vi "Set Aircraft GPS.vi"(7 "Aircraft ID":u8, 8 "Error In":errorcluster, 11 "Aircraft Att Data IN":T1) -> (0 "Error Out":errorcluster, 3 "Aircraft Att Data Out":T1)   [LabVIEW 2014]
uses:
  Controls/Aircraft GPS Data.ctl
  Controls/GPS Fix Type.ctl
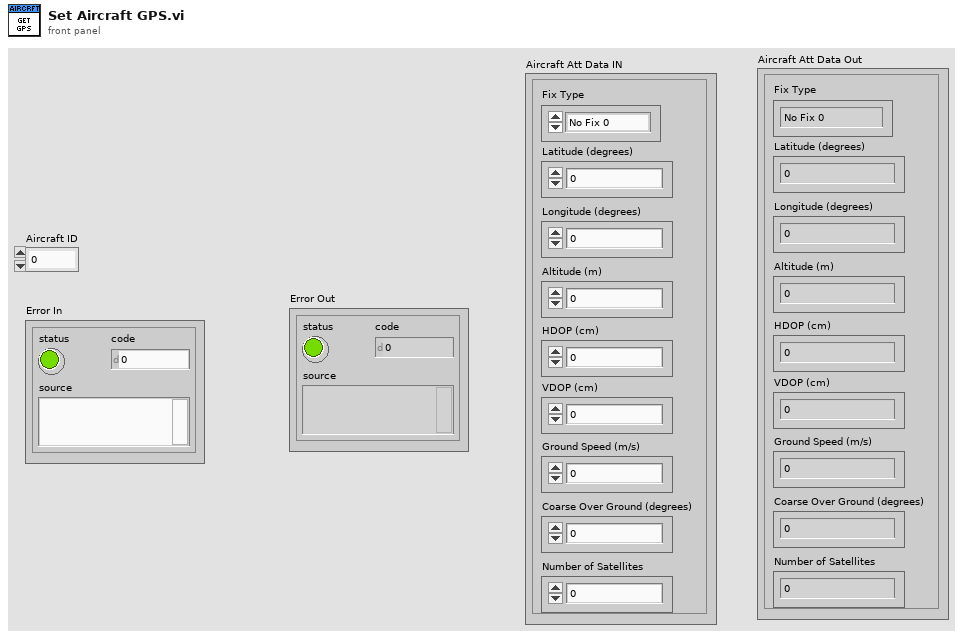
[diagram p1: front panel]
types:
  T1 = typedef "Aircraft GPS Data.ctl" = cluster{"Latitude (degrees)":dbl, "Longitude (degrees)":dbl, "Altitude (m)":dbl, "Fix Type":T2, "HDOP (cm)":u16, "VDOP (cm)":u16, "Ground Speed (m/s)":dbl, "Coarse Over Ground (degrees)":u16, "Number of Satellites":u8}
  T2 = typedef "GPS Fix Type.ctl" = enum16{"No Fix 0", "No Fix 1", "2D Fix", "3D Fix", "DGPS", "RTK"}
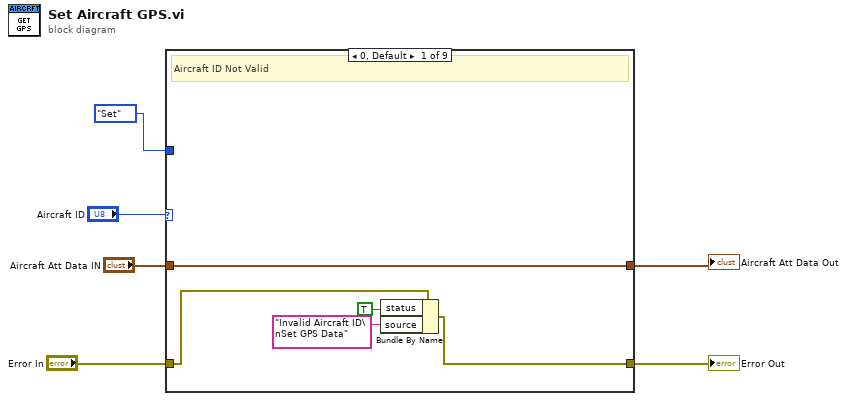
[diagram p0: block diagram]
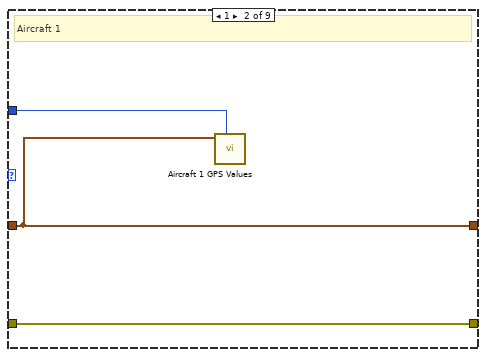
[diagram p2: hidden frame]
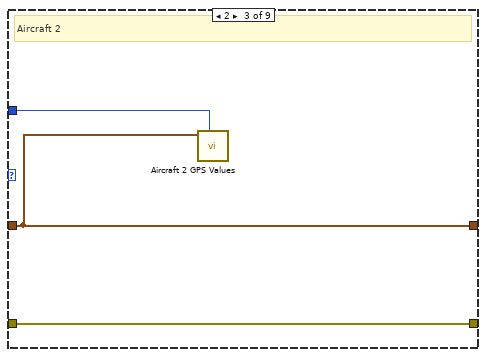
[diagram p3: hidden frame]
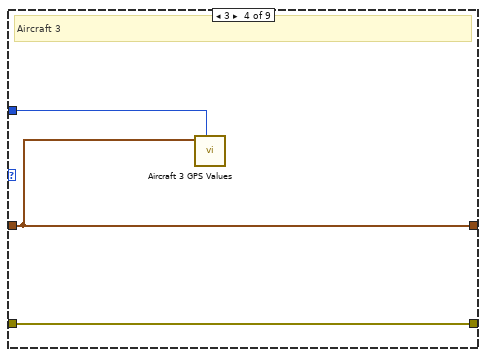
[diagram p4: hidden frame]
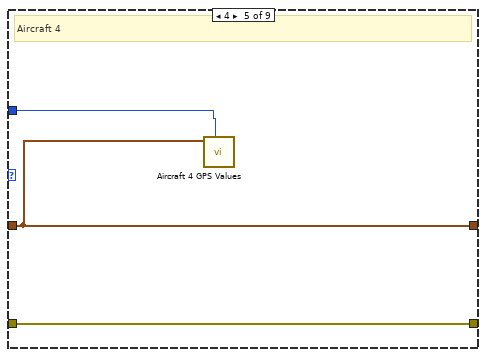
[diagram p5: hidden frame]
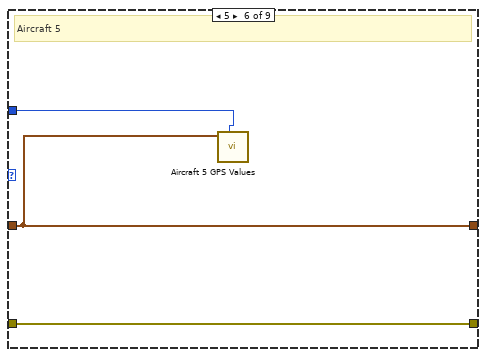
[diagram p6: hidden frame]
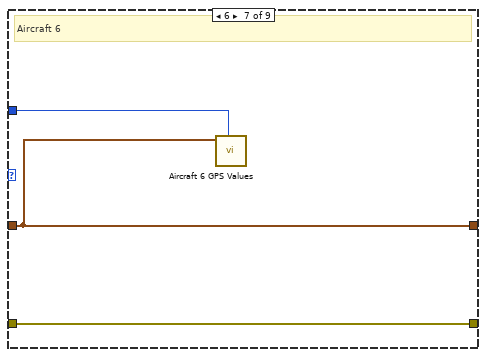
[diagram p7: hidden frame]
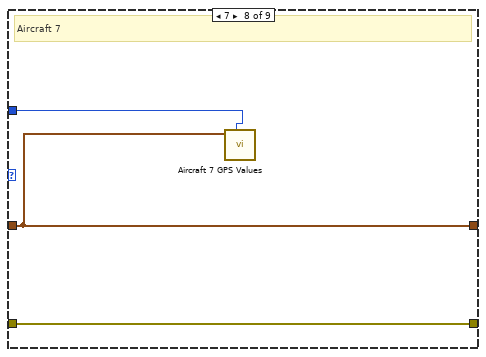
[diagram p8: hidden frame]
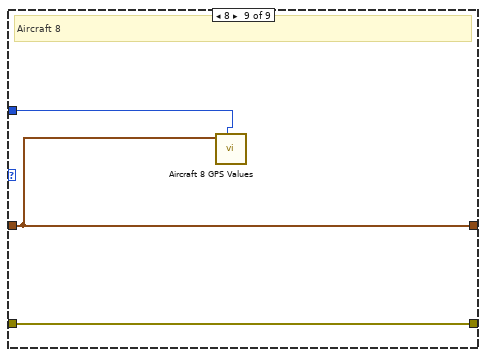
[diagram p9: hidden frame]
diagram:
  n1 = case shown="0, Default" "Aircraft ID" {
    tunnel: [w10 w14 w17 w20 w23 w26 w29 w32 w35] -> w5
    tunnel: "Error In" -> [w11 w14 w17 w20 w23 w26 w29 w32 w35]
    tunnel: enum16{"Get", "Set"}."Set" ("Method") -> [_ w13 w16 w19 w22 w25 w28 w31 w34]
    tunnel: "Aircraft Att Data IN" -> [w7 w12 w15 w18 w21 w24 w27 w30 w33]
    tunnel: [w7 w12 w15 w18 w21 w24 w27 w30 w33] -> w1
    frame 0, Default {
      # "Aircraft ID Not Valid"
      n2 = Bundle By Name(cluster=w11, "status"=TRUE, "source"="Invalid Aircraft ID\nSet GPS Data") -> (w10:errorcluster)
    }
    frame 1 {
      # "Aircraft 1"
      n3 = call "Aircraft 1 GPS Values .vi"("Method"=w13, "Aircraft GPS Data In"=w12) -> ()  [unwired: 9 in, 1 out]
    }
    frame 2 {
      # "Aircraft 2"
      n4 = call "Aircraft 2 GPS Values .vi"("Method"=w16, "Aircraft GPS Data In"=w15) -> ()  [unwired: 9 in, 1 out]
    }
    frame 3 {
      # "Aircraft 3"
      n5 = call "Aircraft 3 GPS Values .vi"("Method"=w19, "Aircraft GPS Data In"=w18) -> ()  [unwired: 9 in, 1 out]
    }
    frame 4 {
      # "Aircraft 4"
      n6 = call "Aircraft 4 GPS Values .vi"("Method"=w22, "Aircraft GPS Data In"=w21) -> ()  [unwired: 9 in, 1 out]
    }
    frame 5 {
      # "Aircraft 5"
      n7 = call "Aircraft 5 GPS Values .vi"("Method"=w25, "Aircraft GPS Data In"=w24) -> ()  [unwired: 9 in, 1 out]
    }
    frame 6 {
      # "Aircraft 6"
      n8 = call "Aircraft 6 GPS Values .vi"("Method"=w28, "Aircraft GPS Data In"=w27) -> ()  [unwired: 9 in, 1 out]
    }
    frame 7 {
      # "Aircraft 7"
      n9 = call "Aircraft 7 GPS Values .vi"("Method"=w31, "Aircraft GPS Data In"=w30) -> ()  [unwired: 9 in, 1 out]
    }
    frame 8 {
      # "Aircraft 8"
      n10 = call "Aircraft 8 GPS Values .vi"("Method"=w34, "Aircraft GPS Data In"=w33) -> ()  [unwired: 9 in, 1 out]
    }
  }
  "Error Out" <- w5
  "Aircraft Att Data Out" <- w1
